vi "Destructor.vi"(8 "error in (no error)":errorcluster, 11 "Mouse in":refnum<class "Keyboard.lvclass">) -> (0 "error out":errorcluster)   [LabVIEW 2021, in "InputDevice.lvlib" / "Keyboard.lvclass"]
uses:
  Keyboard.lvclass
  <vilib>/Utility/inputDevices.llb/closeKeyboard.vi
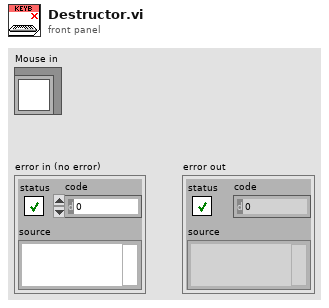
[diagram p1: front panel]
types:
  T1 = typedef "Keyboard.lvclass/data.ctl" = cluster{"DeviceID":refnum<k1>, "Key Pressed":refnum<user-event>, "KeyPressedEvents":refnum<event-registration>, "StopNotifier":refnum<notifier>}
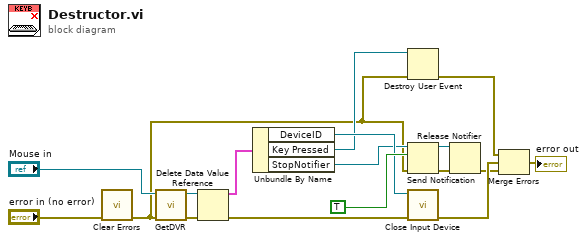
[diagram p0: block diagram]
diagram:
  n1 = call <vilib>:"Clear Errors.vi"("error in (no error)"="error in (no error)") -> ("error out"=w1:errorcluster)  [unwired: 5 in, 1 out]
  n2 = call "GetDVR.vi"("error in (no error)"=w1, "Mouse"="Mouse in") -> ("error out"=w9:errorcluster, "DVR"=w15:refnum<data-value>)  [unwired: 8 in]
  n3 = Delete Data Value Reference(data value reference=w15, error in=w9) -> (data value=w14:T1, error out=w8:errorcluster)
  n4 = Unbundle By Name(w14) -> ("DeviceID"=w13:refnum<k1>, "Key Pressed"=w7:refnum<user-event>, "StopNotifier"=w6:refnum<notifier>)
  n5 = Destroy User Event(user event=w7, error in=w1) -> (error out=w5:errorcluster)
  n6 = Send Notification(notification=TRUE, notifier=w6, error in (no error)=w1) -> (notifier out=w10:refnum<notifier>, error out=w11:errorcluster)
  n7 = call-poly <vilib>:"Close Input Device.vi"("error in (no error)"=w8, "device ID"=w13) -> ("error out"=w4:errorcluster)  [unwired: 8 in]
  n8 = Release Notifier(notifier=w10, error in (no error)=w11) -> (error out=w3:errorcluster)  [unwired: 1 in, 2 out]
  n9 = Merge Errors(w5, w4, w3) -> (→"error out":errorcluster)
